vi "Set AOs.vi"() -> ()   [LabVIEW 2019]
panel:
  in  "stop":bool
  in  "AO5":dbl
  in  "AO4":dbl
  in  "AO3":dbl
  in  "AO2":dbl
  in  "AO1":dbl
  in  "AO0":dbl
  out "error out 2":errorcluster
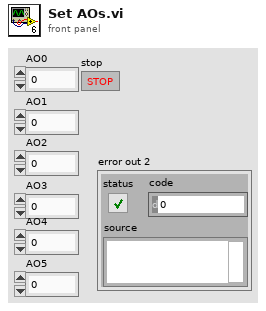
[diagram p1: front panel]
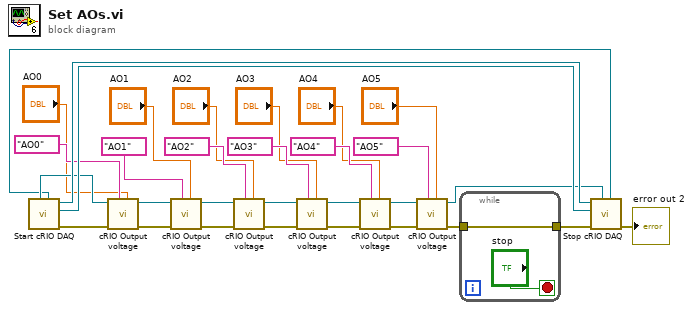
[diagram p0: block diagram]
diagram:
  n1 = call "Start cRIO DAQ.vi"() -> ("error out"=w28:errorcluster, "vi reference"=w30:refnum<vi>, "application reference"=w31:refnum<vi>, "DAQ_AI_Reader endpoint"=w27:refnum<k21>, "DAQ_CMD_Writer endpoint"=w29:refnum<k21>)  [unwired: 7 in]
  n2 = call "cRIO Output voltage.vi"("Voltage"="AO0", "AO Channel"="AO0", "error in (no error)"=w28, "DAQ_CMD_Writer endpoint"=w29) -> ("error out"=w19:errorcluster, "DAQ_CMD_Writer endpoint out"=w14:refnum<k21>)  [unwired: 6 in]
  n3 = call "cRIO Output voltage.vi"("Voltage"="AO1", "AO Channel"="AO1", "error in (no error)"=w19, "DAQ_CMD_Writer endpoint"=w14) -> ("error out"=w18:errorcluster, "DAQ_CMD_Writer endpoint out"=w13:refnum<k21>)  [unwired: 6 in]
  n4 = call "cRIO Output voltage.vi"("Voltage"="AO2", "AO Channel"="AO2", "error in (no error)"=w18, "DAQ_CMD_Writer endpoint"=w13) -> ("error out"=w17:errorcluster, "DAQ_CMD_Writer endpoint out"=w12:refnum<k21>)  [unwired: 6 in]
  n5 = call "cRIO Output voltage.vi"("Voltage"="AO3", "AO Channel"="AO3", "error in (no error)"=w17, "DAQ_CMD_Writer endpoint"=w12) -> ("error out"=w16:errorcluster, "DAQ_CMD_Writer endpoint out"=w11:refnum<k21>)  [unwired: 6 in]
  n6 = call "cRIO Output voltage.vi"("Voltage"="AO4", "AO Channel"="AO4", "error in (no error)"=w16, "DAQ_CMD_Writer endpoint"=w11) -> ("error out"=w15:errorcluster, "DAQ_CMD_Writer endpoint out"=w10:refnum<k21>)  [unwired: 6 in]
  n7 = call "cRIO Output voltage.vi"("Voltage"="AO5", "AO Channel"="AO5", "error in (no error)"=w15, "DAQ_CMD_Writer endpoint"=w10) -> ("error out"=w2:errorcluster, "DAQ_CMD_Writer endpoint out"=w9:refnum<k21>)  [unwired: 6 in]
  n8 = while {
    tunnel: w2 -> [w32]
    tunnel: [w32] -> w1
    stop <- "stop" stop-if-true
  }
  n9 = call "Stop cRIO DAQ.vi"("DAQ_AI_Reader endpoint"=w27, "DAQ_CMD_Writer endpoint"=w9, "error in (no error)"=w1, "VI reference"=w30, "application reference"=w31) -> ("error out"=→"error out 2":errorcluster)  [unwired: 6 in]
